vi "Block Write Scaled Value To Raw.vi"(1 "Scaling Constants":T1, 2 "dbl Scaled Value":dbl[](array[numeric])) -> (7 "u16 Raw Value":u16[](array[numeric]))   [LabVIEW 2021]
uses:
  <vilib>/myRIO/Common/Instrument Driver Framework/Utilities/typedefs/Analog Scaling Constants.ctl
panel:
  # "Converts scaled dbl values to raw ADC u16 values based on the scaling constants."
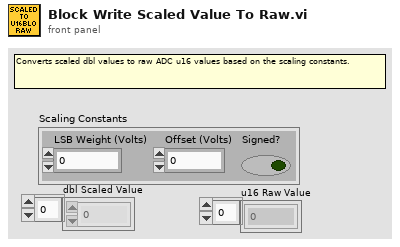
[diagram p1: front panel]
types:
  T1 = typedef "Analog Scaling Constants.ctl" = cluster{"LSB Weight (Volts)":dbl, "Offset (Volts)":dbl, "Signed?":bool}
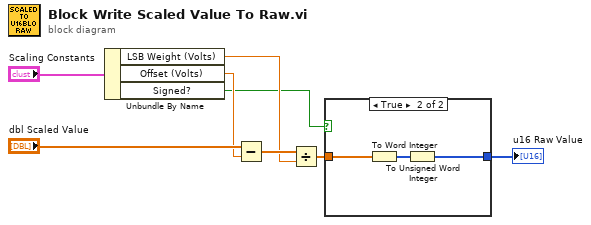
[diagram p0: block diagram]
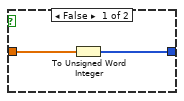
[diagram p2: hidden frame]
diagram:
  n1 = Unbundle By Name("Scaling Constants") -> ("LSB Weight (Volts)"=w4:dbl, "Offset (Volts)"=w6:dbl, "Signed?"=w1:bool)
  n2 = Subtract(x="dbl Scaled Value", y=w6) -> (x-y=w5:dbl[])
  n3 = Divide(x=w5, y=w4) -> (x/y=w3:dbl[])
  n4 = case shown="True" w1 {
    tunnel: w3 -> [w10 w13]
    tunnel: [w9 w11] -> w2
    frame False {
      n5 = To Unsigned Word Integer(number=w10) -> (unsigned 16bit integer=w9:u16[])
    }
    frame True {
      n6 = To Word Integer(number=w13) -> (16bit integer=w12:i16[])
      n7 = To Unsigned Word Integer(number=w12) -> (unsigned 16bit integer=w11:u16[])
    }
  }
  "u16 Raw Value" <- w2
